vi "方程编辑1.vi"(8 "X":dbl, 9 "B":dbl, 10 "C":dbl, 11 "A":dbl) -> (3 "输出变量":dbl)   [LabVIEW 2018]
uses:
  <vilib>/express/express arith-compare/Formula/XNode/ExpressFormulaBlockNode.xnode
panel:
  out "结果":dbl
  in  "X 2":dbl
  in  "C 2":dbl
  in  "B 2":dbl
  in  "A 2":dbl
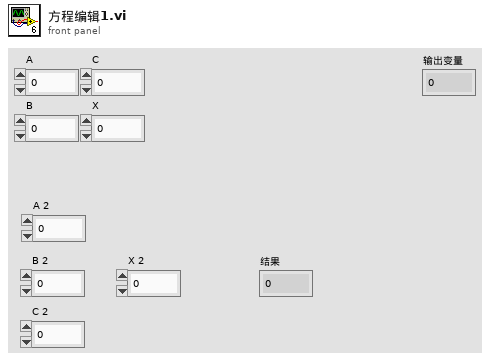
[diagram p1: front panel]
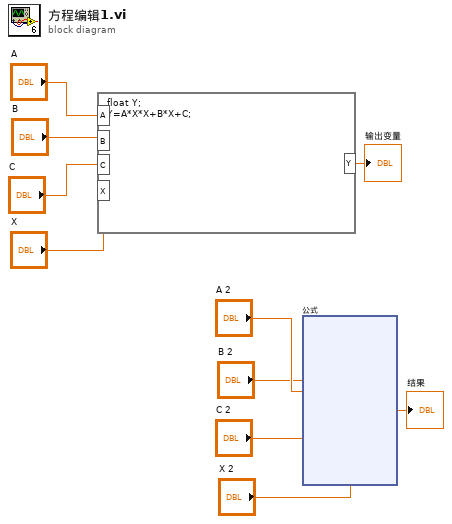
[diagram p0: block diagram]
diagram:
  n1 = formula code="float Y;\nY=A*X*X+B*X+C;"("A"="A", "B"="B", "C"="C", "X"="X") -> ("Y"=→"输出变量":dbl)
  n2 = xnode "公式"("A"="A 2", "B"="B 2", "C"="C 2", "X"="X 2") -> ("结果"=→"结果":dbl)  [unwired: 1 in, 1 out]
